vi "Set AP Sx Parameter.vi"(8 "error in (no error)":errorcluster caption="错误输入（无错误）", 9 "para2":i32, 10 "asicBitsName":i32, 11 "asicHandle":i32) -> (0 "error out":errorcluster caption="错误输出", 3 "function return":i32)   [LabVIEW 2020]
doc: "extern int SetAPSxParameter (int asicHandle, int asicBitsName, IN ...);"
uses:
  APSx.dll/APSx.dll
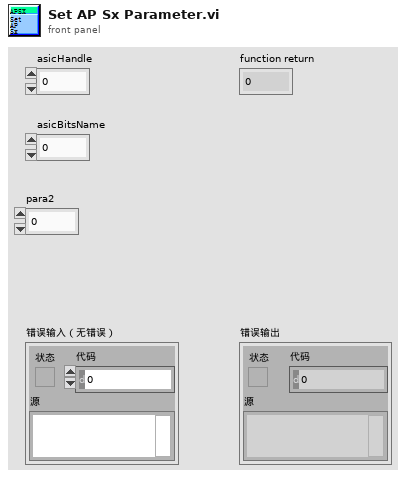
[diagram p1: front panel]
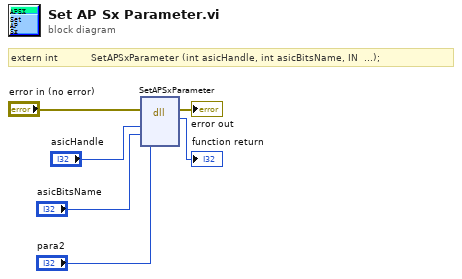
[diagram p0: block diagram]
diagram:
  # "extern int           SetAPSxParameter (int asicHandle, int asicBitsName, IN  ...);"
  n1 = dll-call lib="PTH2gabs CUsersFengDesktop传感器对中台传感器对中台labviewSourcesAPSx.dllAPSx.*" fn="SetAPSxParameter"(error in="error in (no error)", "asicHandle"="asicHandle", "asicBitsName"="asicBitsName", "para2"="para2") -> (error out=→"error out":errorcluster, "返回类型"=→"function return":i32)  [unwired: 5 in, 1 out]
